vi "LVAPT-GIT-Status.vi"(11 "path":path) -> ()   [LabVIEW 2019]
uses:
  <vilib>/Hampel Software Engineering/Git API/Git API/GIT-api.lvclass/GIT-api.ctl
  <vilib>/Hampel Software Engineering/Git API/Git API/Accessors/GIT-Set Working Dir.vi
  <vilib>/Hampel Software Engineering/Git API/Git API/GIT-api.lvclass
panel:
  out "Staged Files":string[](array[string])
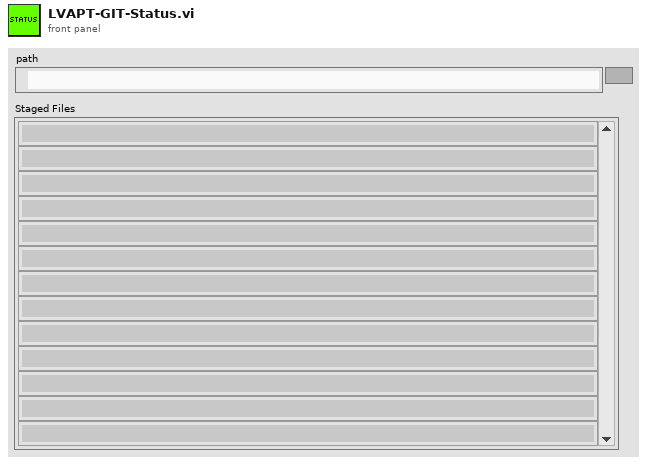
[diagram p1: front panel]
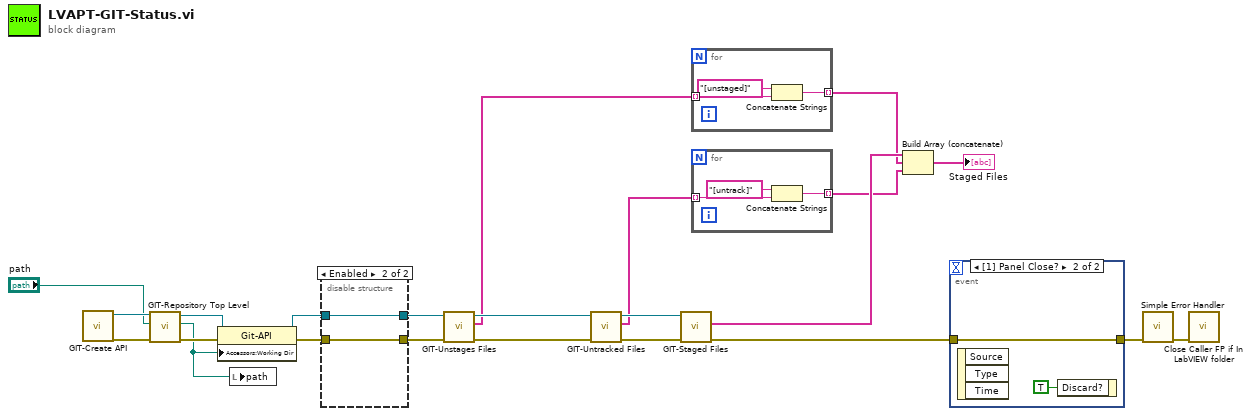
[diagram p0: block diagram]
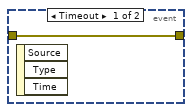
[diagram p2: hidden frame]
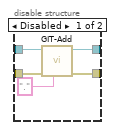
[diagram p3: hidden frame]
diagram:
  n1 = call <vilib>:"GIT-Create API.vi"() -> ("error out"=w20:errorcluster, "git-api out"=w21:refnum<class "GIT-api.lvclass">)  [unwired: 10 in]
  n2 = call <vilib>:"GIT-Repository Top Level.vi"("error in"=w20, "Current Path"="path", "git-api in"=w21) -> ("error out"=w23:errorcluster, "Repo Top Level Path"=w16:path, "git-api out"=w22:refnum<class "GIT-api.lvclass">)  [unwired: 6 in]
  n3 = property class="Git-API"(reference=w22, error in=w23, "Accessors:Working Dir"=w16) -> (reference out=w18:refnum<class "GIT-api.lvclass">, error out=w19:errorcluster)
  n4 = local write "path"(w16) -> ()
  n5 = disable-structure shown="Enabled" {
    disable-tunnel: w19 -> [w28 w29]
    disable-tunnel: w18 -> [w27 w30]
    disable-tunnel: [w25 w30] -> w14
    disable-tunnel: [w24 w29] -> w11
    frame Disabled {
      n6 = call <vilib>:"GIT-Add.vi"("param"=".", "error in"=w28, "git-api in"=w27) -> ("error out"=w24:errorcluster, "git-api out"=w25:refnum<class "GIT-api.lvclass">)  [unwired: 6 in, 1 out]
    }
    frame Enabled {
    }
  }
  n7 = call <vilib>:"GIT-Unstages Files.vi"("error in"=w11, "Git-API in"=w14) -> ("error out"=w12:errorcluster, "Unstaged Files"=w8:string[], "Git-API out"=w13:refnum<class "GIT-api.lvclass">)  [unwired: 7 in]
  n8 = call <vilib>:"GIT-Untracked Files.vi"("error in"=w12, "Git-API in"=w13) -> ("error out"=w10:errorcluster, "Untracked Files"=w7:string[], "Git-API out"=w9:refnum<class "GIT-api.lvclass">)  [unwired: 7 in]
  n9 = call <vilib>:"GIT-Staged Files.vi"("error in"=w10, "Git-API in"=w9) -> ("error out"=w2:errorcluster, "Staged Files"=w15:string[])  [unwired: 7 in, 1 out]
  n10 = for {
    tunnel: w8 -> [w33] mode=indexing
    tunnel: [w31] -> w5 mode=indexing
    n11 = Concatenate Strings("[unstaged]" ("string"), w33) -> (w31:string)
  }
  n12 = for {
    tunnel: w7 -> [w36] mode=indexing
    tunnel: [w34] -> w4 mode=indexing
    n13 = Concatenate Strings("[untrack]" ("string"), w36) -> (w34:string)
  }
  n14 = Build Array (concatenate)(w15, w5, w4) -> (→"Staged Files":string[])
  n15 = event shown="[1] Panel Close?" {
    selector: _ -> [_ _]
    dyn-events: _ -> [_ _]
    timeout: _ -> [_ _]
    tunnel: w2 -> [w37 w39]
    tunnel: [w37 w39] -> w1
    event Timeout {
      n16 = event-data() -> ()  [unwired: 1 in, 3 out]
    }
    event Panel Close? {
      n17 = event-data() -> ()  [unwired: 1 in, 3 out]
      n18 = event-data("Discard?"=TRUE) -> ()  [unwired: 1 in, 1 out]
    }
  }
  n19 = call <vilib>:"Simple Error Handler.vi"("error in (no error)"=w1) -> ("error out"=w3:errorcluster)  [unwired: 4 in, 4 out]
  n20 = call "Close Caller FP if In LabVIEW folder.vi"("error in (no error)"=w3) -> ()  [unwired: 10 in, 1 out]
